vi "checkForFirstLineAttributes.vi"(8 "error in (no error)":errorcluster, 10 "XML In":string, 11 "ReadAttribute In":refnum<class "XMLAttributeParser.lvclass">) -> (0 "error out":errorcluster, 2 "firstLineAttributeFound":bool, 3 "ReadAttribute Out":refnum<class "XMLAttributeParser.lvclass">)   [LabVIEW 2016, in "XML.lvlib" / "XMLAttributeParser.lvclass"]
doc: "This method checks the first line if there are any attributes by looking for \\sAttributeType=\"AttributeValue\""
uses:
  <userlib>/Common/XML/XMLAttributeParser/XMLAttributeParser.lvclass
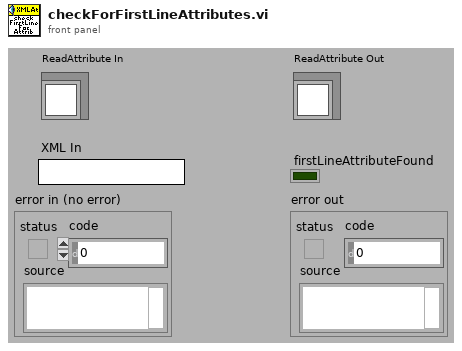
[diagram p1: front panel]
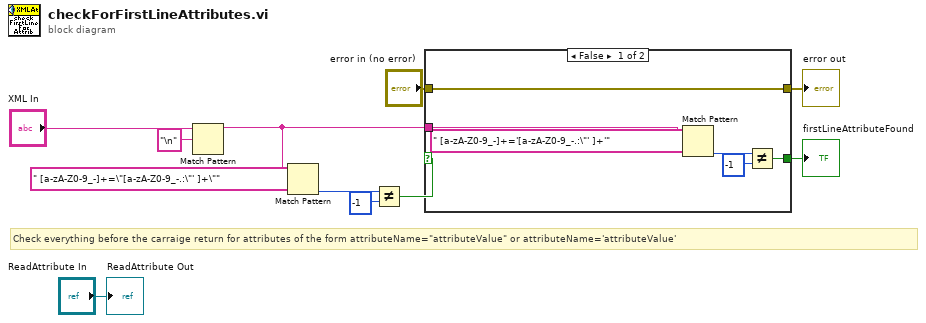
[diagram p0: block diagram]
diagram:
  # "Check everything before the carraige return for attributes of the form attributeName=\"attributeValue\" or attributeName='attributeValue'"
  n1 = Match Pattern(string="XML In", regular expression="\n") -> (before substring=w5:string)  [unwired: 1 in, 3 out]
  n2 = Match Pattern(string=w5, regular expression=" [a-zA-Z0-9_-]+=\"[a-zA-Z0-9_-.:\"' ]+\"") -> (offset past match=w9:i32)  [unwired: 1 in, 3 out]
  n3 = Not Equal?(x=w9, y=-1) -> (x != y?=w4:bool)
  n4 = case shown="False" w4 {
    selector: w4 -> [_ w19]
    tunnel: w5 -> [w15 _]
    tunnel: [w13 w19] -> w3
    tunnel: "error in (no error)" -> [w12 w18]
    tunnel: [w12 w18] -> w1
    frame False {
      n5 = Match Pattern(string=w15, regular expression=" [a-zA-Z0-9_-]+='[a-zA-Z0-9_-.:\"' ]+'") -> (offset past match=w14:i32)  [unwired: 1 in, 3 out]
      n6 = Not Equal?(x=w14, y=-1) -> (x != y?=w13:bool)
    }
    frame True {
    }
  }
  "firstLineAttributeFound" <- w3
  "error out" <- w1
  "ReadAttribute Out" <- "ReadAttribute In"
